vi "Initialise.vi"(8 "Error In":errorcluster, 9 "Environment Options":T1, 10 "Path Overrides":T2={"Webview2 Native"=path "C:/Users/kleins/Desktop/webview2/microsoft.web.webview2.1.0.1370.28/build/native", "Edge Application"=path "", "User Data"=path ""}, 11 "object in":refnum<class "WebView.lvclass">) -> (0 "Error Out":errorcluster, 3 "object out":refnum<class "WebView.lvclass">)   [LabVIEW 2024, in "WebView.lvclass"]
uses:
  WebView.lvclass
  WebView.lvclass/WebView.ctl
  <vilib>/sklein/WebView2/Libs/Microsoft.Web.WebView2.Core.dll
  Resources--cluster.ctl
  Events--cluster.ctl
  Navigation Complete Event Data--cluster.ctl
  Source Changed Event Data--cluster.ctl
  Navigation Start Event Data--cluster.ctl
  <vilib>/sklein/WebView2/Libs/Microsoft.Web.WebView2.WinForms.dll
  Paths-cluster.ctl
  Core Envrionment Options--cluster.ctl
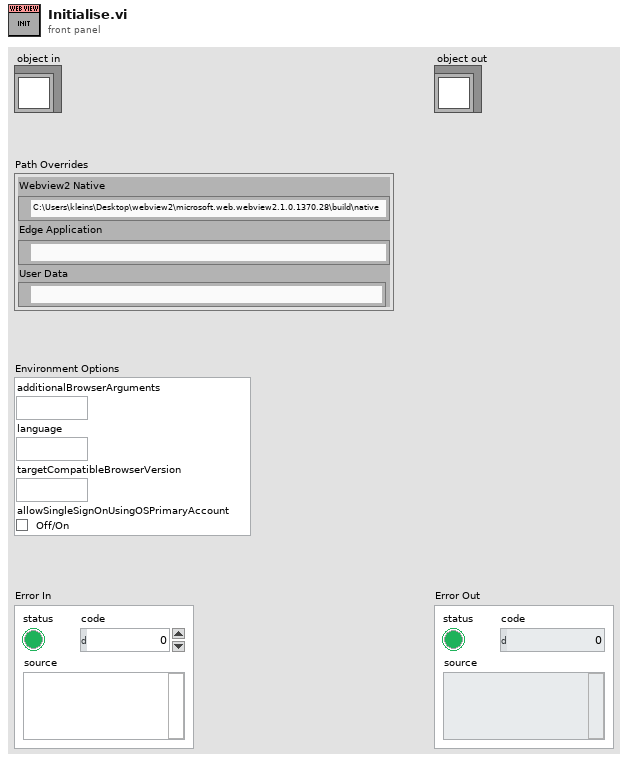
[diagram p1: front panel]
types:
  T1 = typedef "WebView.lvclass/Core Envrionment Options--cluster.ctl" = cluster{"additionalBrowserArguments":string, "language":string, "targetCompatibleBrowserVersion":string, "allowSingleSignOnUsingOSPrimaryAccount":bool}
  T2 = typedef "WebView.lvclass/Paths-cluster.ctl" = cluster{"Webview2 Native":path, "Edge Application":path, "User Data":path}
  T3 = typedef "WebView.lvclass/Navigation Start Event Data--cluster.ctl" = cluster{"AdditionalAllowedFrameAncestors":string, "Cancel":bool, "IsRedirected":bool, "IsUserInitiated":bool, "NavigationId":u64, "NavigationKind":i32, "RequestHeaders":refnum<k24>, "Uri":string}
  T4 = typedef "WebView.lvclass/Navigation Complete Event Data--cluster.ctl" = cluster{"HttpStatusCode":i32, "IsSuccess?":bool, "NavigationId":u64, "WebErrorStatus":i32}
  T5 = cluster{"Source":string, "WebMessageAsJson":string}
  T6 = typedef "WebView.lvclass/Events--cluster.ctl" = cluster{"Navigation Complete Event":refnum<user-event>, "Source Changed Event":refnum<user-event>, "Document Title Changed Event":refnum<user-event>, "Status Bar Text Changed":refnum<user-event>, "Web Message Received":refnum<user-event>, "Window Close Requested":refnum<user-event>, "DOM Loaded":refnum<user-event>, "Navigation Started Event":refnum<user-event>}
  T7 = typedef "WebView.lvclass/Source Changed Event Data--cluster.ctl" = cluster{"Source":string, "IsNewDocument":bool}
  T8 = typedef "WebView.lvclass/Resources--cluster.ctl" = cluster{"WebView2":refnum<k24>, "Webview2 Core":refnum<k24>, "event callback":refnum<k27>, "Environment":refnum<k24>}
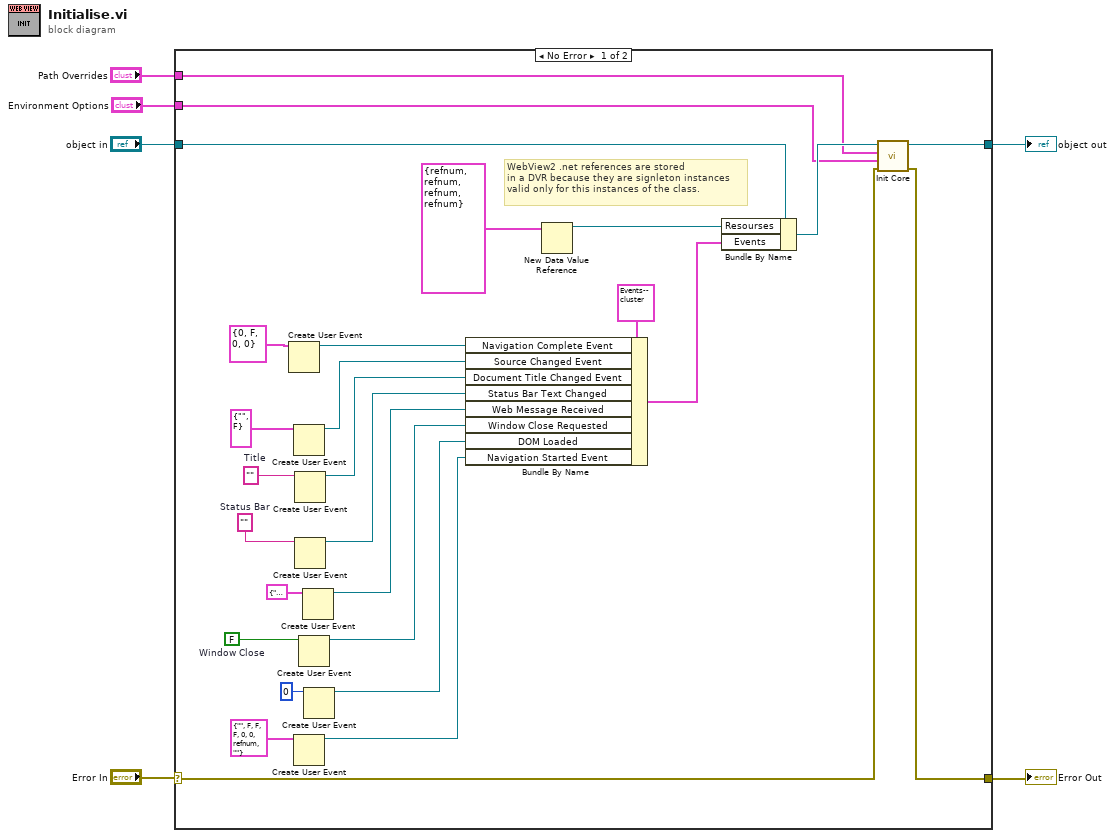
[diagram p0: block diagram]
diagram:
  n1 = case shown="No Error" "Error In" {
    selector: "Error In" -> [w10 w34]
    tunnel: "object in" -> [w33 w35]
    tunnel: [w11 w35] -> w5
    tunnel: [w9 w34] -> w3
    tunnel: "Path Overrides" -> [w8 _]
    tunnel: "Environment Options" -> [w7 _]
    frame No Error {
      w21 = FALSE  # Window Close
      w24 = ""  # Status Bar
      w29 = ""  # Title
      # "WebView2 .net references are stored \nin a DVR because they are signleton instances\nvalid only for this instances of the class."
      n2 = Create User Event(user event datatype=T4 {"HttpStatusCode"=0, "IsSuccess?"=FALSE, "NavigationId"=0, "WebErrorStatus"=0} ("output cluster")) -> (user event=w26:refnum<user-event>)  [unwired: 1 in, 1 out]
      n3 = Create User Event(user event datatype=T7 {"Source"="", "IsNewDocument"=FALSE} ("Source")) -> (user event=w25:refnum<user-event>)  [unwired: 1 in, 1 out]
      n4 = Create User Event(user event datatype=T3 {"AdditionalAllowedFrameAncestors"="", "Cancel"=FALSE, "IsRedirected"=FALSE, "IsUserInitiated"=FALSE, "NavigationId"=0, "NavigationKind"=0, "RequestHeaders"=refnum, "Uri"=""} ("Nav Started Event")) -> (user event=w15:refnum<user-event>)  [unwired: 1 in, 1 out]
      n5 = Create User Event(user event datatype=w29) -> (user event=w27:refnum<user-event>)  [unwired: 1 in, 1 out]
      n6 = Create User Event(user event datatype=w24) -> (user event=w23:refnum<user-event>)  [unwired: 1 in, 1 out]
      n7 = Create User Event(user event datatype=w21) -> (user event=w20:refnum<user-event>)  [unwired: 1 in, 1 out]
      n8 = Create User Event(user event datatype=T5 {"Source"="", "WebMessageAsJson"=""} ("output cluster")) -> (user event=w22:refnum<user-event>)  [unwired: 1 in, 1 out]
      n9 = Create User Event(user event datatype=u64 0 ("NavigationId")) -> (user event=w18:refnum<user-event>)  [unwired: 1 in, 1 out]
      n10 = Bundle By Name(cluster=T6 {"Navigation Complete Event"=refnum, "Source Changed Event"=refnum, "Document Title Changed Event"=refnum, "Status Bar Text Changed"=refnum, "Web Message Received"=refnum, "Window Close Requested"=refnum, "DOM Loaded"=refnum, "Navigation Started Event"=refnum} ("Cluster"), "Navigation Complete Event"=w26, "Source Changed Event"=w25, "Document Title Changed Event"=w27, "Status Bar Text Changed"=w23, "Web Message Received"=w22, "Window Close Requested"=w20, "DOM Loaded"=w18, "Navigation Started Event"=w15) -> (w13:T6)
      n11 = New Data Value Reference(data value=T8 {"WebView2"=refnum, "Webview2 Core"=refnum, "event callback"=refnum, "Environment"=refnum}) -> (data value reference=w31:refnum<data-value>)  [unwired: 1 in, 1 out]
      n12 = Bundle By Name(cluster=w33, "Resourses"=w31, "Events"=w13) -> (w12:refnum<class "WebView.lvclass">)
      n13 = call "Init Core.vi"("Error In"=w10, "Environment Options"=w7, "Path Overrides"=w8, "object in"=w12) -> ("Error Out"=w9:errorcluster, "object out"=w11:refnum<class "WebView.lvclass">)  [unwired: 6 in]
    }
    frame Error {
    }
  }
  "object out" <- w5
  "Error Out" <- w3
